vi "Tab.vi"(5 "Tab Control In":enum32{"Page 1", "Page 2", "Page 3"}(tab)) -> (2 "Tab Control Out":enum32{"Page 1", "Page 2", "Page 3", "Page 4"}(tab))   [LabVIEW 2011]
panel:
  in  "String 3":string
  in  "Numeric 3":dbl format="%.2f"
  in  "Numeric 4":dbl format="%.2f"
  out "String 4":string
  in  "Boolean":bool
  in  "String":string
  in  "Numeric":dbl format="%.2f"
  in  "Numeric 2":dbl format="%.2f"
  out "String 2":string
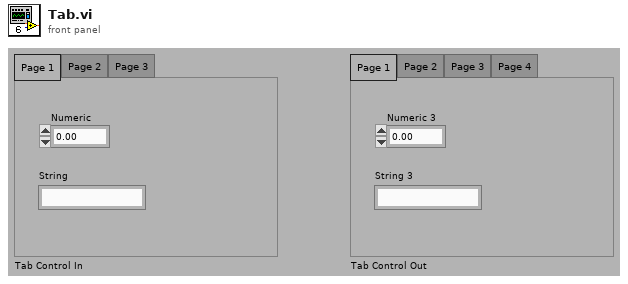
[diagram p1: front panel]
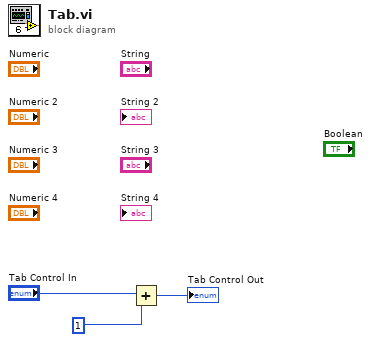
[diagram p0: block diagram]
diagram:
  n1 = Add(x="Tab Control In", y=1) -> (x+y=→"Tab Control Out":u32)
